vi "Initialize.vi"(8 "error in (no error)":errorcluster, 11 "[V] Sys Cfg Base in":refnum<class "[V] Sys Cfg Base.lvclass">) -> (0 "error out":errorcluster, 3 "[V] Sys Cfg Base out":refnum<class "[V] Sys Cfg Base.lvclass">)   [LabVIEW 2023, in "[V] Sys Cfg Base.lvlib" / "[V] Sys Cfg Base.lvclass"]
uses:
  [V] Sys Cfg Base.lvclass
  [V] Sys Cfg Base.lvclass/[V] Sys Cfg Base.ctl
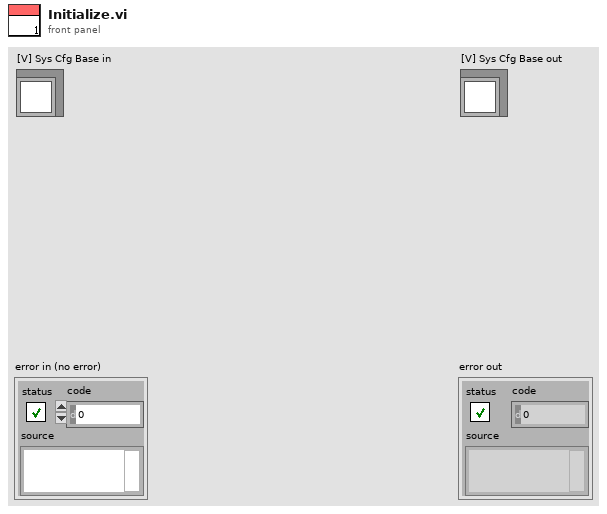
[diagram p1: front panel]
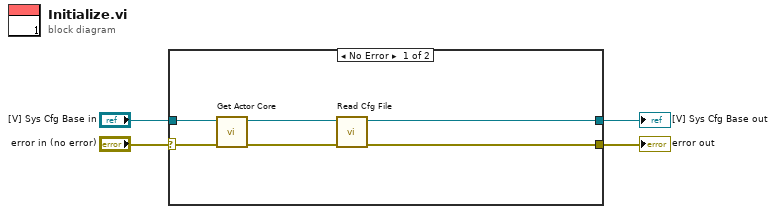
[diagram p0: block diagram]
diagram:
  n1 = case shown="No Error" "error in (no error)" {
    selector: "error in (no error)" -> [w10 w12]
    tunnel: [w6 w12] -> w3
    tunnel: [w7 w11] -> w1
    tunnel: "[V] Sys Cfg Base in" -> [w5 w11]
    frame No Error {
      n2 = call "Get Actor Core.vi"("error in (no error)"=w10, "[V] Sys Cfg Base in"=w5) -> ("error out"=w9:errorcluster, "[V] Sys Cfg Base out"=w8:refnum<class "[V] Sys Cfg Base.lvclass">)  [unwired: 8 in]
      n3 = call-dynamic "Read Cfg File.vi"("error in (no error)"=w9, "[V] Sys Cfg Base in"=w8) -> ("error out"=w6:errorcluster, "[V] Sys Cfg Base out"=w7:refnum<class "[V] Sys Cfg Base.lvclass">)  [unwired: 8 in]
    }
    frame Error {
    }
  }
  "error out" <- w3
  "[V] Sys Cfg Base out" <- w1
